vi "RegisterWriteTest (FPGA).vi"() -> ()   [LabVIEW 2009]
uses:
  <vilib>/eio/EIONode/EIONode.xnode
  <vilib>/rvi/eio/nirviEIOImplementation/nirviEIOImplementation.xnode
  <vilib>/rvi/eio/common/nirviEmuTemplateMethod_noerrors.vi
  <vilib>/rvi/eio/common/nirviEmuClasses.ctl
panel:
  in  "Count(uSec)":u32=800
  in  "Point":cluster{"X":i32, "Y":i32, "Z":i32} {"Z" format="%x"; "Y" format="%x"; "X" format="%x"}
  in  "UpdatesPerPoint":u32
  in  "stop 2":bool
  in  "Write Points":bool
  in  "P":bool
  in  "stop":bool
  in  "Pause":u32
  in  "WriteSize":enum16{"1", "2", "4"}(ring)
  in  "Divider":u32=2
  in  "NumRegs":i16=10
  in  "Update IO time":u32=20
  in  "Register  Values":cluster{"Address":u8, "Value":u32}[](array[cluster])=[{"Address"=0, "Value"=240}, {"Address"=1, "Value"=13762592}, {"Address"=2, "Value"=32768}, {"Address"=3, "Value"=8413952}, {"Address"=4, "Value"=858993459}, {"Address"=5, "Value"=0}, {"Address"=6, "Value"=1023}, {"Address"=7, "Value"=257}, {"Address"=8, "Value"=21}, {"Address"=10, "Value"=858993459}, {"Address"=0, "Value"=240}, {"Address"=0, "Value"=0}, {"Address"=0, "Value"=0}, {"Address"=0, "Value"=0}, {"Address"=0, "Value"=0}, {"Address"=0, "Value"=0}, {"Address"=0, "Value"=0}, {"Address"=0, "Value"=0}, {"Address"=0, "Value"=0}, {"Address"=0, "Value"=0}] {"Address" format="%x"; "Value" format="%x"}
  in  "Write Registers":bool
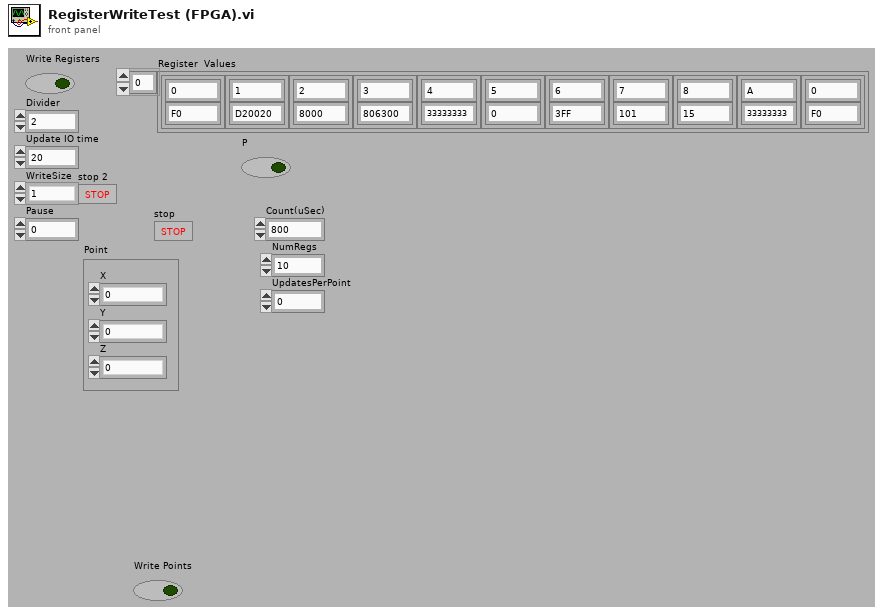
[diagram p1: front panel]
types:
  T1 = typedef "nirviEmuClasses.ctl" = enum16{"IO Read", "IO Write", "Method", "Property Read", "Property Write"}
  T2 = cluster{"XHPstart":u32, "XHPend":u32, "XLPstart":u32, "XLPend":u32, "YHPstart":u32, "YHPend":u32, "YLPstart":u32, "YLPend":u32, "RR":u32, "FR":u32}
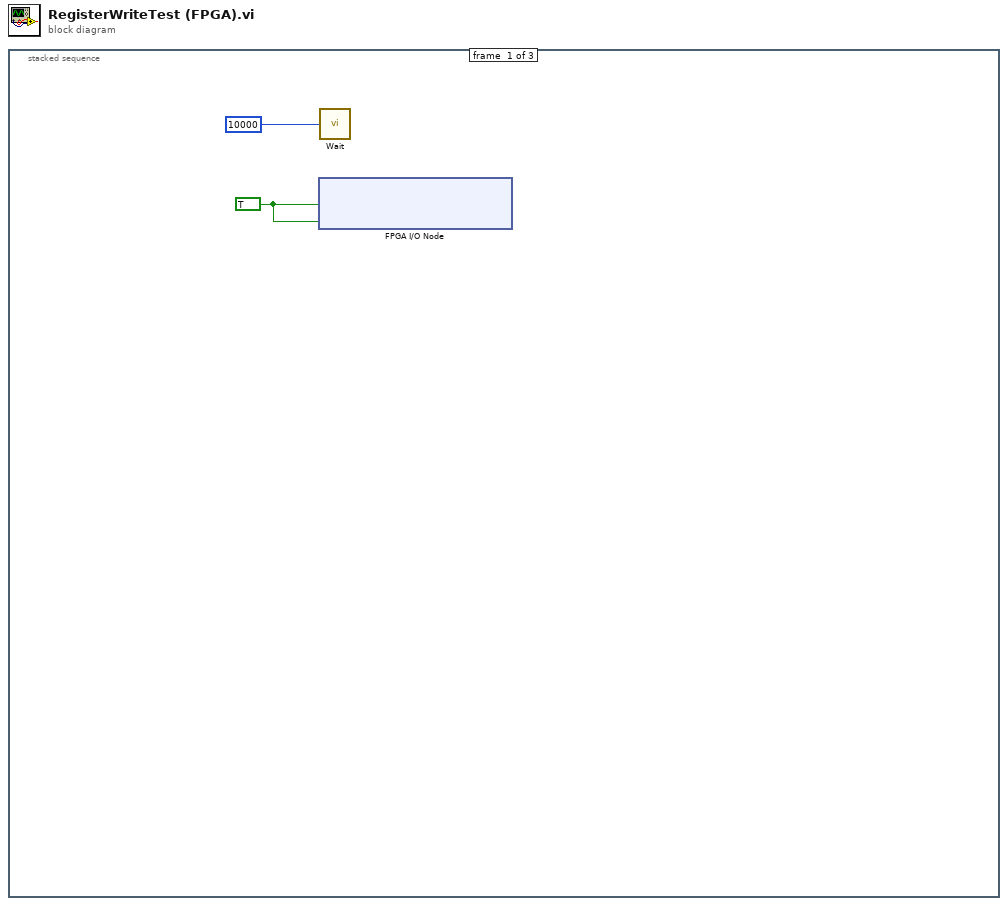
[diagram p0: block diagram]
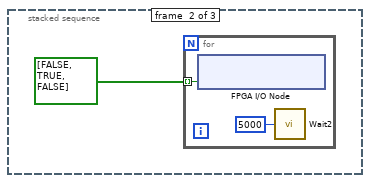
[diagram p2: hidden frame]
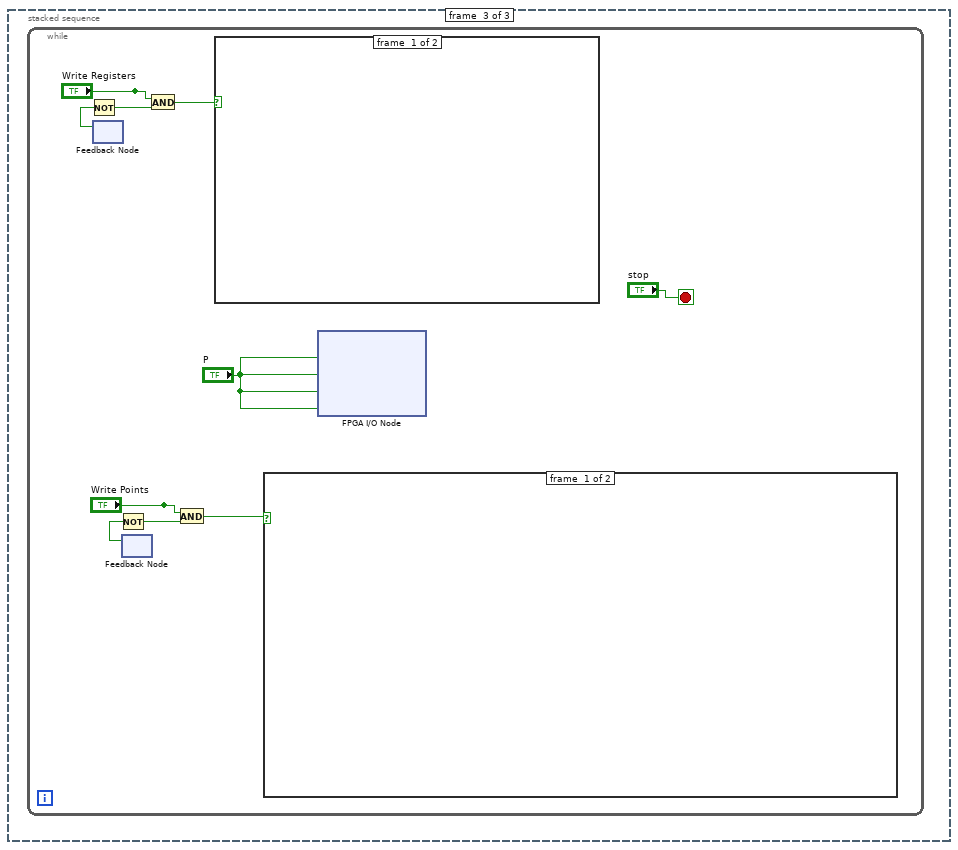
[diagram p3: hidden frame]
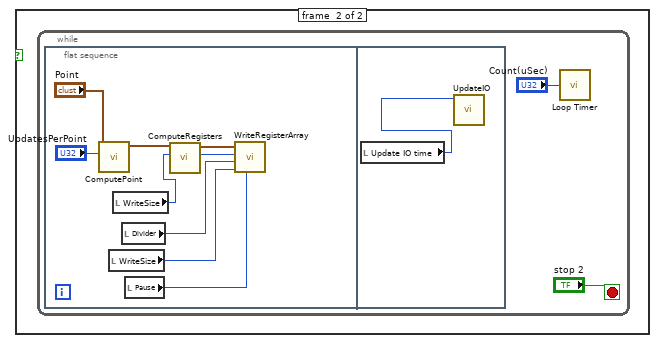
[diagram p4: hidden frame]
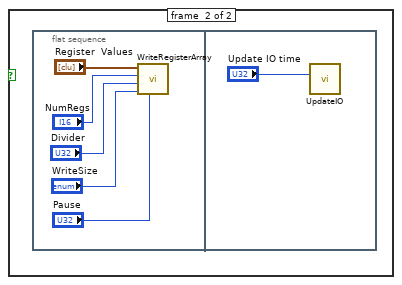
[diagram p5: hidden frame]
diagram:
  n1 = stacked-sequence {
    frame #0 {
      w1 = TRUE ("IO Module\\DDCA_DIO0-7_WE")
      n2 = xnode "FPGA I/O Node"("IO Module\\DDCA_DIO0-7_WE"=w1, "IO Module\\DDCA_DIO8-15_WE"=w1) -> ()  [unwired: 2 in, 2 out]
      n3 = call "Wait"("Count(uSec)"=u32 10000) -> ()  [unwired: 1 out]
    }
    frame #1 {
      n4 = for {
        tunnel: bool[] [FALSE, TRUE, FALSE] -> [w26] mode=indexing
        n5 = xnode "FPGA I/O Node"("IO Module\\RESET"=w26) -> ()  [unwired: 1 in, 1 out]
        n6 = call "Wait2"("Count(uSec)"=u32 5000) -> ()  [unwired: 1 out]
      }
    }
    frame #2 {
      n7 = while {
        stop <- "stop" stop-if-true
        n8 = feedback #1() -> (w48:bool)  [unwired: 1 in]
        n9 = Not(x=w48) -> (.not. x?=w46:bool)
        n10 = feedback #2() -> (w42:bool)  [unwired: 1 in]
        n11 = Not(x=w42) -> (.not. x?=w40:bool)
        n12 = And(x="Write Registers", y=w46) -> (x .and. y?=w45:bool)
        n13 = And(x="Write Points", y=w40) -> (x .and. y?=w39:bool)
        n14 = case shown="True" w45 {
          frame #0 {
          }
          frame #1 {
            n15 = flat-sequence {
              frame #0 {
                n16 = call "WriteRegisterArray.vi"("Pause"="Pause", "WriteSize"="WriteSize", "SclkDivider"="Divider", "NumReg"="NumRegs", "Register  Values"="Register  Values") -> ()  [unwired: 7 in]
              }
              frame #1 {
                n17 = call "UpdateIO.vi"("Count(ticks)"="Update IO time") -> ()  [unwired: 11 in]
              }
            }
          }
        }
        n18 = case shown="True" w39 {
          frame #0 {
          }
          frame #1 {
            n19 = while {
              stop <- "stop 2" stop-if-true
              n20 = flat-sequence {
                frame #0 {
                  n21 = call "ComputePoint.vi"("UpdatesPerPoint"="UpdatesPerPoint", "Point"="Point") -> ("output cluster"=w59:T2)  [unwired: 9 in]
                  n22 = local read "WriteSize"() -> (w55:enum16{"1", "2", "4"})
                  n23 = local read "WriteSize"() -> (w58:enum16{"1", "2", "4"})
                  n24 = local read "Divider"() -> (w54:u32)
                  n25 = local read "Pause"() -> (w53:u32)
                  n26 = call "ComputeRegisters.vi"("WriteSize"=w58, "coordinates"=w59) -> ("Numeric"=w56:i16, "Register Writes"=w57:cluster{"Address":u8, "Value":u32}[])  [unwired: 8 in]
                  n27 = call "WriteRegisterArray.vi"("Pause"=w53, "WriteSize"=w55, "SclkDivider"=w54, "NumReg"=w56, "Register  Values"=w57) -> ()  [unwired: 7 in]
                }
                frame #1 {
                  n28 = local read "Update IO time"() -> (w60:u32)
                  n29 = call "UpdateIO.vi"("Count(ticks)"=w60) -> ()  [unwired: 11 in]
                }
              }
              n30 = call "Loop Timer"("Count(uSec)"="Count(uSec)") -> ()  [unwired: 1 out]
            }
          }
        }
        n31 = xnode "FPGA I/O Node"("IO Module\\P0"="P", "IO Module\\P1"="P", "IO Module\\P2"="P", "IO Module\\P3"="P") -> ()  [unwired: 4 in, 4 out]
      }
    }
  }
